vi "Acumulador2.vi"(11 "Numeric in":dbl) -> (3 "Numeric":dbl)   [LabVIEW 2018]
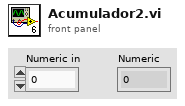
[diagram p1: front panel]
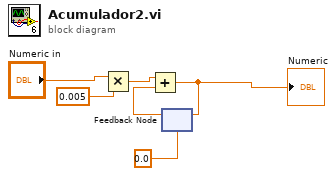
[diagram p0: block diagram]
diagram:
  n1 = Multiply(x="Numeric in", y=0.005) -> (x*y=w2:dbl)
  n2 = feedback #1(0.0) -> (w5:dbl)
  n3 = Add(x=w2, y=w5) -> (x+y=w1:dbl)
  "Numeric" <- w1
  n4 = feedback-in #1(w1) -> ()
